vi "Construct Terminal Value Binding.vi"(10 "Ctl Refnum":refnum<vi>, 11 "TerminalValueBinding In":refnum<class "TerminalValueBinding.lvclass">) -> (0 "error out":errorcluster, 3 "TerminalValueBinding Out":refnum<class "TerminalValueBinding.lvclass">)   [LabVIEW 2017, in "TerminalValueBinding.lvclass"]
doc: "<License>\nCopyright © 2017 Composed Systems, LLC | All rights reserved\nwww.composed.io\n\nAuthor: Ethan Stern <ethan.stern@composed.io>\n\nThis software is provided \"AS IS\" WITHOUT WARRANTIES, either express or implied, AND IS FOR EDUCATIONAL PURPOSES ONLY.\n</License>"
uses:
  <vilib>/gpm_packages/@cs/transport/Source/Concrete/TerminalValueBinding/TerminalValueBinding.lvclass
  <vilib>/gpm_packages/@cs/transport/Source/Concrete/TerminalValueBinding/TerminalValueBinding.lvclass/TerminalValueBinding.ctl
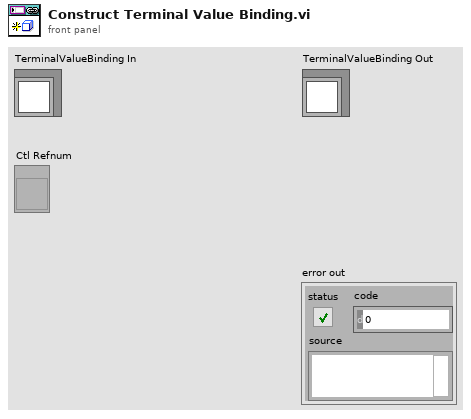
[diagram p1: front panel]
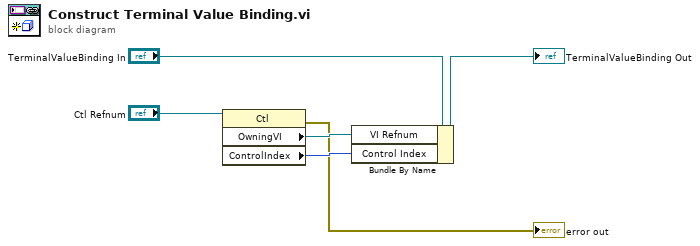
[diagram p0: block diagram]
diagram:
  n1 = property class="Ctl"(reference="Ctl Refnum") -> (error out=→"error out":errorcluster, "OwningVI"=w4:refnum<vi>, "ControlIndex"=w3:i32)  [unwired: 1 in, 1 out]
  n2 = Bundle By Name(cluster="TerminalValueBinding In", "VI Refnum"=w4, "Control Index"=w3) -> (→"TerminalValueBinding Out":refnum<class "TerminalValueBinding.lvclass">)
